vi "P9P14_Temp_Merge_Cluster.vi"(1 "P9-P14 T-Cluster -Control":T2 {"Approach" items=["Fast Settle", "No O'Shoot"]}, 2 "P9-P14 T-Cluster-Status":T1 {"Temperature\nStatus" items=["TemperatureUnknown"=0, "Stable"=1, "Tracking"=2, "Near"=5, "Chasing"=6, "Filling"=7, "Standby"=10, "Disabled"=13, "ImpedanceNotFunction"=14, "TempFailure"=15]}) -> (0 "P9-P14 T-Cluster":T3 {"Temperature\nStatus" items=["TemperatureUnknown"=0, "Stable"=1, "Tracking"=2, "Near"=5, "Chasing"=6, "Filling"=7, "Standby"=10, "Disabled"=13, "ImpedanceNotFunction"=14, "TempFailure"=15]; "Approach" items=["Fast Settle", "No O'Shoot"]})   [LabVIEW 2019]
uses:
  PPMS/P9P14-TCluster.ctl
  PPMS/P9P14-TCluster-Control.ctl
  PPMS/P9P14-TCluster-Status.ctl
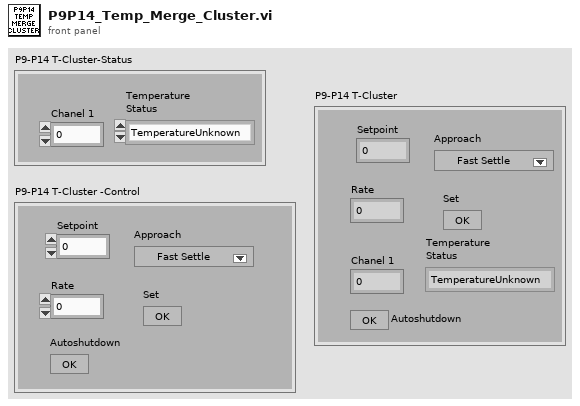
[diagram p1: front panel]
types:
  T1 = typedef "P9P14-TCluster-Status.ctl" = cluster{"Chanel 1":dbl, "Temperature\nStatus":i32}
  T2 = typedef "P9P14-TCluster-Control.ctl" = cluster{"Setpoint":dbl, "Rate":dbl, "Approach":u16, "Set":bool, "Autoshutdown":bool}
  T3 = typedef "P9P14-TCluster.ctl" = cluster{"Setpoint":dbl, "Rate":dbl, "Chanel 1":dbl, "Approach":u16, "Set":bool, "Temperature\nStatus":i32, "Autoshutdown":bool}
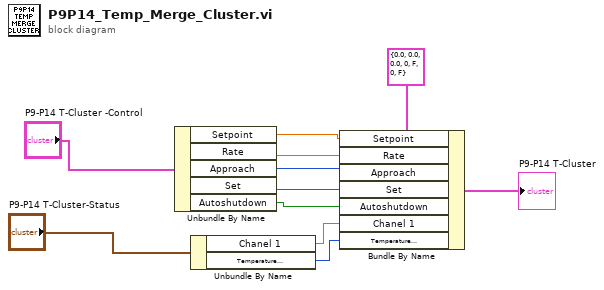
[diagram p0: block diagram]
diagram:
  n1 = Unbundle By Name("P9-P14 T-Cluster -Control") -> ("Setpoint"=w8:dbl, "Rate"=w7:dbl, "Approach"=w6:u16, "Set"=w5:bool, "Autoshutdown"=w1:bool)
  n2 = Unbundle By Name("P9-P14 T-Cluster-Status") -> ("Chanel 1"=w2:dbl, "Temperature\nStatus"=w3:i32)
  n3 = Bundle By Name(cluster=T3 {"Setpoint"=0.0, "Rate"=0.0, "Chanel 1"=0.0, "Approach"=0, "Set"=FALSE, "Temperature\nStatus"=0, "Autoshutdown"=FALSE} ("P9-P14 T-Cluster"), "Setpoint"=w8, "Rate"=w7, "Approach"=w6, "Set"=w5, "Autoshutdown"=w1, "Chanel 1"=w2, "Temperature\nStatus"=w3) -> (→"P9-P14 T-Cluster":T3)
